vi "Execute.vi"(8 "error in (no error)":errorcluster, 10 "System In":refnum<class "bt_System.lvclass">, 11 "Node in":refnum<class "bt_Decorator.lvclass">) -> (0 "error out":errorcluster, 1 "Status":T1, 2 "System Out":refnum<class "bt_System.lvclass">, 3 "Node out":refnum<class "bt_Decorator.lvclass">)   [LabVIEW 2021, in "BT.lvlib" / "bt_Decorator.lvclass"]
uses:
  bt_Decorator.lvclass
  abs_Node/Status.ctl
  abs_System/bt_System.lvclass
  bt_Decorator.lvclass/bt_Decorator.ctl
  abs_Node/bt_Node.lvclass
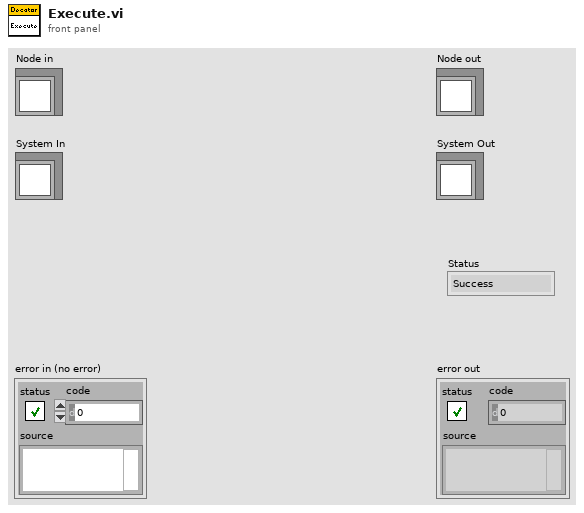
[diagram p1: front panel]
types:
  T1 = typedef "BT.lvlib/bt_Node.lvclass/Status.ctl" = enum16{"Success", "Failure", "Running"}
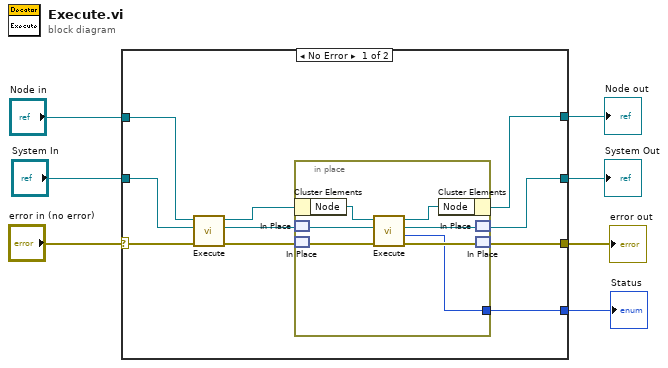
[diagram p0: block diagram]
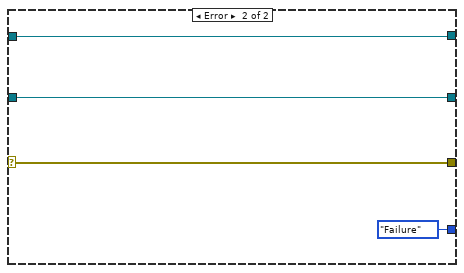
[diagram p2: hidden frame]
diagram:
  n1 = case shown="No Error" "error in (no error)" {
    selector: "error in (no error)" -> [w17 w26]
    tunnel: "System In" -> [w16 w27]
    tunnel: "Node in" -> [w15 w28]
    tunnel: [w11 w26] -> w4
    tunnel: [w10 w28] -> w3
    tunnel: [w9 w27] -> w2
    tunnel: [w8 Status."Failure" ("Status")] -> w1
    frame No Error {
      n2 = call-parent "Execute.vi"("error in (no error)"=w17, "System In"=w16, "Node in"=w15) -> ("error out"=w12:errorcluster, "System Out"=w13:refnum<class "bt_System.lvclass">, "Node out"=w14:refnum<class "bt_Decorator.lvclass">)  [unwired: 5 in, 1 out]
      n3 = in-place {
        in-place-border: [w18] -> w8
        n4 = in-place-cluster #1(w14) -> ("Node"=w24:refnum<class "bt_Node.lvclass">)
        n5 = in-place-match #2(w13) -> (w21:refnum<class "bt_System.lvclass">)
        n6 = in-place-match #3(w12) -> (w20:errorcluster)
        n7 = call-dynamic "Execute.vi"("error in (no error)"=w20, "System In"=w21, "Node in"=w24) -> ("error out"=w19:errorcluster, "Status"=w18:T1, "System Out"=w22:refnum<class "bt_System.lvclass">, "Node out"=w23:refnum<class "bt_Node.lvclass">)  [unwired: 5 in]
        n8 = in-place-cluster #1("Node"=w23) -> (w10:refnum<class "bt_Decorator.lvclass">)
        n9 = in-place-match #2(w22) -> (w9:refnum<class "bt_System.lvclass">)
        n10 = in-place-match #3(w19) -> (w11:errorcluster)
      }
    }
    frame Error {
    }
  }
  "error out" <- w4
  "Node out" <- w3
  "Status" <- w1
  "System Out" <- w2
